vi "RIOcardStorage.vi"(8 "Error in":errorcluster, 9 "Channel Settings":T4[][](array[typedef]), 10 "Card Settings":T1 {"Sample Rate" format="%#_3p"}, 11 "Tree DVR in":refnum<data-value>) -> (0 "error out":errorcluster)   [LabVIEW 2014]
uses:
  Controls/RIOSettingsChannelSettings.ctl
  <vilib>/MDSplus/Classes/Tree_Class/Tree.lvclass
  Controls/RIOSettingsCardSettingsArray.ctl
  Controls/RIOSettingsCardSettings.ctl
  <vilib>/userdefined/High Color/nirio_resource_hc.ctl
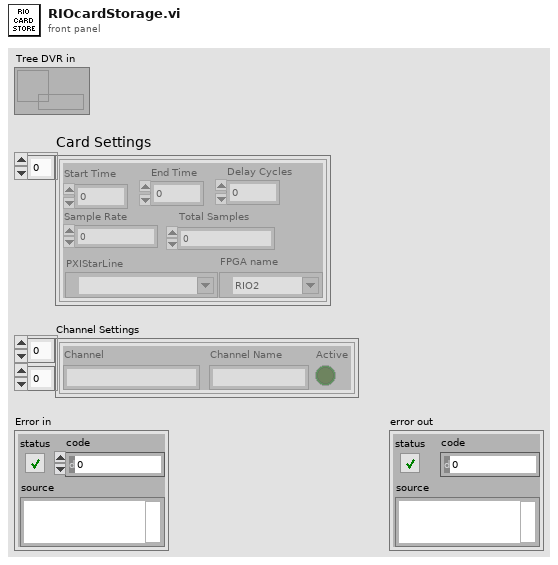
[diagram p1: front panel]
types:
  T1 = typedef "RIOSettingsCardSettingsArray.ctl" = T2[]
  T2 = typedef "RIOSettingsCardSettings.ctl" = cluster{"Start Time":dbl, "End Time":dbl, "Sample Rate":dbl, "Total Samples":u64, "PXIStarLine":tag, "Delay Cycles":u64, "FPGA name":T3}
  T3 = typedef "nirio_resource_hc.ctl" = tag
  T4 = typedef "RIOSettingsChannelSettings.ctl" = cluster{"Channel Name":string, "Active":bool, "Channel":string}
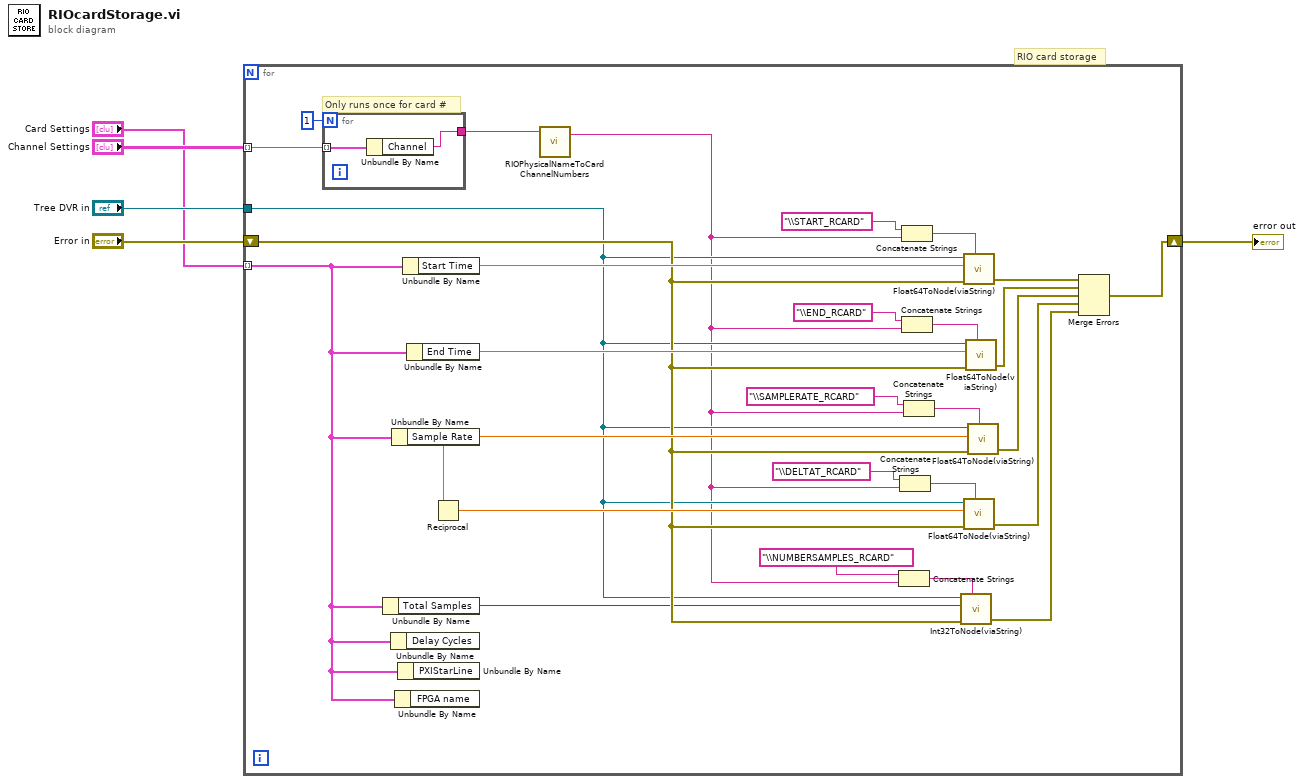
[diagram p0: block diagram]
diagram:
  # "RIO card storage"
  n1 = for {
    tunnel: "Card Settings" -> [w33] mode=indexing
    shift-right: [w27] -> w2
    shift-left: "Error in" -> [w11]
    tunnel: "Channel Settings" -> [w32] mode=indexing
    tunnel: "Tree DVR in" -> [w10]
    # "Only runs once for card #"
    n2 = for {
      N: 1 -> [_]
      tunnel: w32 -> [w35] mode=indexing
      tunnel: [w34] -> w7
      n3 = Unbundle By Name(w35) -> ("Channel"=w34:string)
    }
    n4 = Unbundle By Name(w33) -> ("Total Samples"=w8:u64)
    n5 = Unbundle By Name(w33) -> ()  [unwired: 1 out]
    n6 = Unbundle By Name(w33) -> ("Sample Rate"=w18:dbl)
    n7 = Unbundle By Name(w33) -> ()  [unwired: 1 out]
    n8 = Unbundle By Name(w33) -> ()  [unwired: 1 out]
    n9 = Unbundle By Name(w33) -> ("Start Time"=w26:dbl)
    n10 = Unbundle By Name(w33) -> ("End Time"=w23:dbl)
    n11 = Reciprocal(x=w18) -> (1/x=w15:dbl)
    n12 = call "RIOPhysicalNameToCardChannelNumbers.vi"("Channel Name"=w7) -> ("Card #"=w6:string)  [unwired: 1 in, 1 out]
    n13 = Concatenate Strings("\\NUMBERSAMPLES_RCARD" ("string"), w6) -> (w13:string)
    n14 = Concatenate Strings("\\DELTAT_RCARD" ("string"), w6) -> (w16:string)
    n15 = Concatenate Strings("\\START_RCARD" ("string"), w6) -> (w29:string)
    n16 = Concatenate Strings("\\END_RCARD" ("string"), w6) -> (w24:string)
    n17 = Concatenate Strings("\\SAMPLERATE_RCARD" ("string"), w6) -> (w20:string)
    n18 = call "Int32ToNode(viaString).vi"("Tree DVR in"=w10, "I32 in"=w8, "error in (no error)"=w11, "NodePath"=w13) -> ("error out"=w9:errorcluster)  [unwired: 1 in, 2 out]
    n19 = call "Float64ToNode(viaString).vi"("Tree DVR in"=w10, "DBL in"=w26, "error in"=w11, "NodePath"=w29) -> ("error out"=w30:errorcluster)  [unwired: 1 in, 2 out]
    n20 = call "Float64ToNode(viaString).vi"("Tree DVR in"=w10, "DBL in"=w15, "error in"=w11, "NodePath"=w16) -> ("error out"=w14:errorcluster)  [unwired: 1 in, 2 out]
    n21 = call "Float64ToNode(viaString).vi"("Tree DVR in"=w10, "DBL in"=w23, "error in"=w11, "NodePath"=w24) -> ("error out"=w22:errorcluster)  [unwired: 1 in, 2 out]
    n22 = call "Float64ToNode(viaString).vi"("Tree DVR in"=w10, "DBL in"=w18, "error in"=w11, "NodePath"=w20) -> ("error out"=w19:errorcluster)  [unwired: 1 in, 2 out]
    n23 = Merge Errors(w30, w22, w19, w14, w9) -> (w27:errorcluster)
  }
  "error out" <- w2
